vi "SPI.vi"() -> ()   [LabVIEW 2021]
uses:
  <instrlib>/niDigital/niDigital.llb/niDigital Burst Pattern (Pass Fail).vi
  <instrlib>/niDigital/niDigital.llb/niDigital Get Site Results Site Numbers.vi
  <instrlib>/niDigital/niDigital.llb/niDigital Selected Function.ctl
panel:
  out "I3C Pass":bool[](array[boolean])
  out "I3C Site":string[](array[string])
  out "I2C Pass":bool[](array[boolean])
  out "I2C Site":string[](array[string])
  in  "error in":errorcluster
  out "error out":errorcluster
  in  "I3C Digital Pattern":refnum<k15>="PXI1Slot2,PXI1Slot3" caption="resource name"
  in  "Simulate?":bool=TRUE
  in  "I2C Pattern":refnum<k15>="PXI1Slot2,PXI1Slot3" caption="resource name"
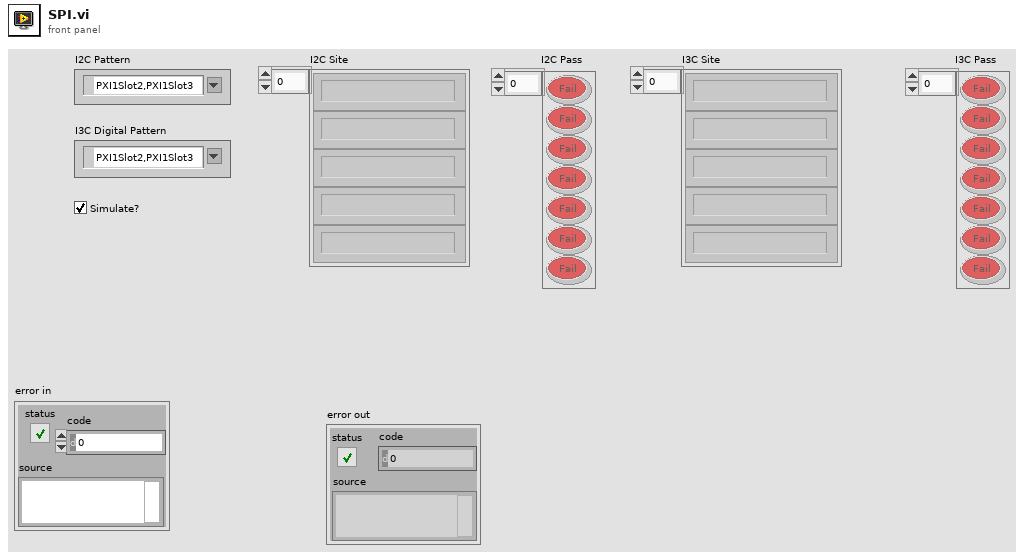
[diagram p1: front panel]
types:
  T1 = typedef "niDigital Selected Function.ctl" = i32
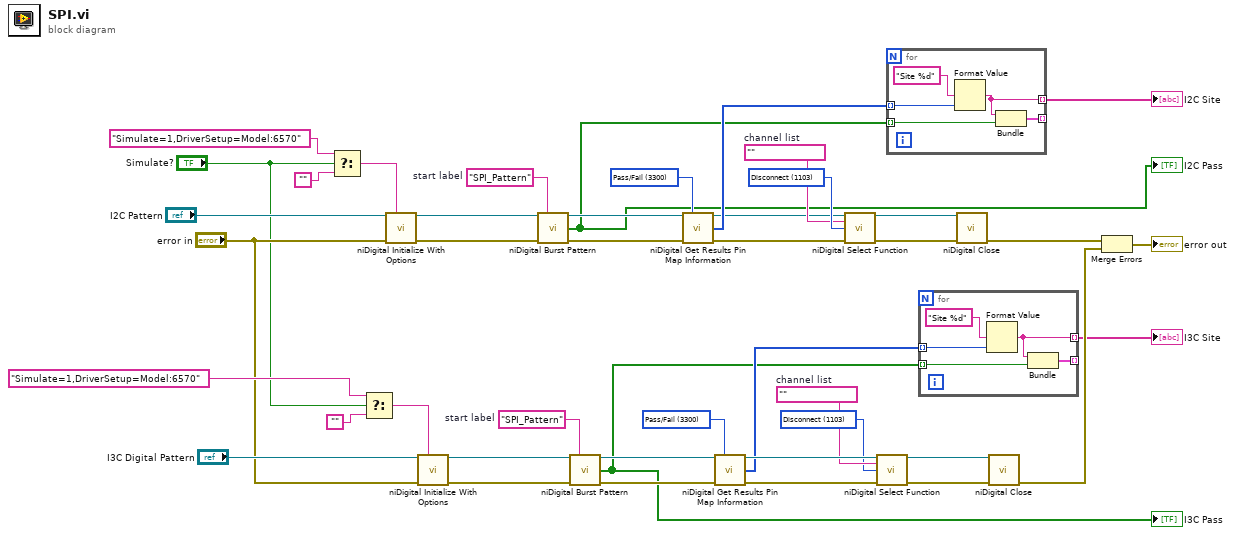
[diagram p0: block diagram]
diagram:
  w16 = ""  # channel list
  w15 = T1 1103 items=["Digital"=1100, "PPMU"=1101, "Off"=1102, "Disconnect"=1103] ("function")
  w10 = "SPI_Pattern"  # start label
  w14 = 3300 items=["Pass/Fail"=3300, "Capture Waveform"=3301] ("site result type")
  w37 = ""  # channel list
  w38 = T1 1103 items=["Digital"=1100, "PPMU"=1101, "Off"=1102, "Disconnect"=1103] ("function")
  w43 = "SPI_Pattern"  # start label
  w39 = 3300 items=["Pass/Fail"=3300, "Capture Waveform"=3301] ("site result type")
  n1 = Select(t="Simulate=1,DriverSetup=Model:6570", s="Simulate?", f="") -> (s? t:f=w31:string)
  n2 = Select(t="Simulate=1,DriverSetup=Model:6570", s="Simulate?", f="") -> (s? t:f=w22:string)
  n3 = call <instrlib>:"niDigital Initialize With Options.vi"("resource name"="I2C Pattern", "option string"=w31, "error in"="error in") -> ("instrument handle"=w28:refnum<k15>, "error out"=w27:errorcluster)  [unwired: 11 in]
  n4 = call <instrlib>:"niDigital Initialize With Options.vi"("resource name"="I3C Digital Pattern", "option string"=w22, "error in"="error in") -> ("instrument handle"=w25:refnum<k15>, "error out"=w26:errorcluster)  [unwired: 11 in]
  n5 = call-poly <instrlib>:"niDigital Burst Pattern.vi"("instrument handle"=w28, "start label"=w43, "error in"=w27) -> ("instrument handle out"=w42:refnum<k15>, "pass"=w3:bool[], "error out"=w41:errorcluster)  [unwired: 10 in]
  "I2C Pass" <- w3
  n6 = call-poly <instrlib>:"niDigital Burst Pattern.vi"("instrument handle"=w25, "start label"=w10, "error in"=w26) -> ("instrument handle out"=w11:refnum<k15>, "pass"=w1:bool[], "error out"=w12:errorcluster)  [unwired: 10 in]
  "I3C Pass" <- w1
  n7 = call-poly <instrlib>:"niDigital Get Results Pin Map Information.vi"("instrument handle"=w42, "site result type"=w39, "error in"=w41) -> ("instrument handle out"=w36:refnum<k15>, "site numbers"=w40:i32[], "error out"=w35:errorcluster)  [unwired: 10 in]
  n8 = call-poly <instrlib>:"niDigital Get Results Pin Map Information.vi"("instrument handle"=w11, "site result type"=w14, "error in"=w12) -> ("instrument handle out"=w17:refnum<k15>, "site numbers"=w13:i32[], "error out"=w18:errorcluster)  [unwired: 10 in]
  n9 = call <instrlib>:"niDigital Select Function.vi"("instrument handle"=w36, "channel list"=w37, "function"=w38, "error in"=w35) -> ("instrument handle out"=w33:refnum<k15>, "error out"=w34:errorcluster)  [unwired: 10 in]
  n10 = call <instrlib>:"niDigital Select Function.vi"("instrument handle"=w17, "channel list"=w16, "function"=w15, "error in"=w18) -> ("instrument handle out"=w20:refnum<k15>, "error out"=w19:errorcluster)  [unwired: 10 in]
  n11 = for {
    tunnel: w3 -> [w48] mode=indexing
    tunnel: [w47] -> _ mode=indexing
    tunnel: w40 -> [w45] mode=indexing
    tunnel: [w44] -> w4 mode=indexing
    n12 = Format Value(format string="Site %d", value (0)=w45) -> (output string=w44:string)  [unwired: 1 in]
    n13 = Bundle("output string"=w44, w48) -> (w47:cluster{"output string":string, bool})  [unwired: 1 in]
  }
  "I2C Site" <- w4
  n14 = for {
    tunnel: w1 -> [w53] mode=indexing
    tunnel: [w52] -> _ mode=indexing
    tunnel: w13 -> [w50] mode=indexing
    tunnel: [w49] -> w2 mode=indexing
    n15 = Format Value(format string="Site %d", value (0)=w50) -> (output string=w49:string)  [unwired: 1 in]
    n16 = Bundle("output string"=w49, w53) -> (w52:cluster{"output string":string, bool})  [unwired: 1 in]
  }
  "I3C Site" <- w2
  n17 = call <instrlib>:"niDigital Close.vi"("instrument handle"=w33, "error in"=w34) -> ("error out"=w9:errorcluster)  [unwired: 13 in]
  n18 = call <instrlib>:"niDigital Close.vi"("instrument handle"=w20, "error in"=w19) -> ("error out"=w7:errorcluster)  [unwired: 13 in]
  n19 = Merge Errors(w9, w7) -> (→"error out":errorcluster)
